vi "ReversedEngineering QueuedStateMachinieMemory.vi"(1 "VIName":string, 2 "StateJumps":string[](array[string]), 5 "error in (no error)":errorcluster, 6 "Action(GetInsertQueuedArrayElementsVI)":T1=enum."GetInsertQueuedArrayElementsVI") -> (15 "StateJumpsOut":string[][](array[string]), 16 "VIName":string, 19 "error out":errorcluster)   [LabVIEW 2020]
uses:
  <resource>/Framework/Providers/Open_GDS/UML/ReversedEngineering/ReversedEngineering QueuedStateMachinMemoryAction.ctl
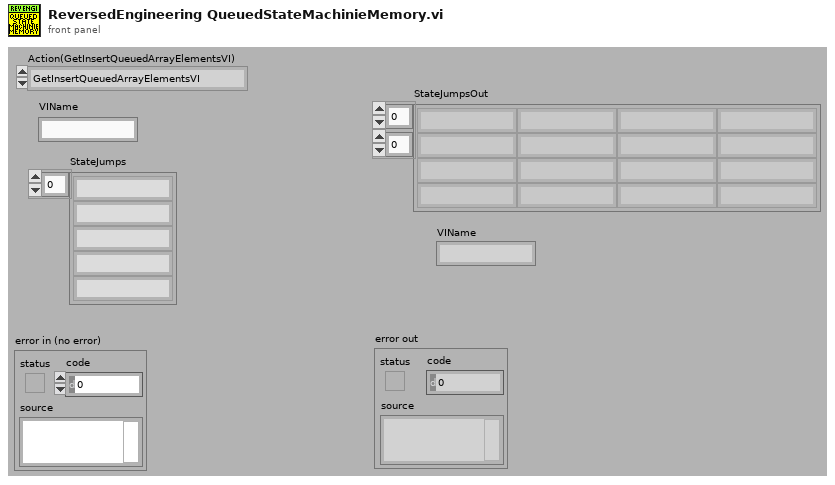
[diagram p1: front panel]
types:
  T1 = typedef "ReversedEngineering QueuedStateMachinMemoryAction.ctl" = enum16{"Initialize", "GetInsertQueuedArrayElementsVI", "SetQueuedStateJumps", "GetQueuedStateJumps"}
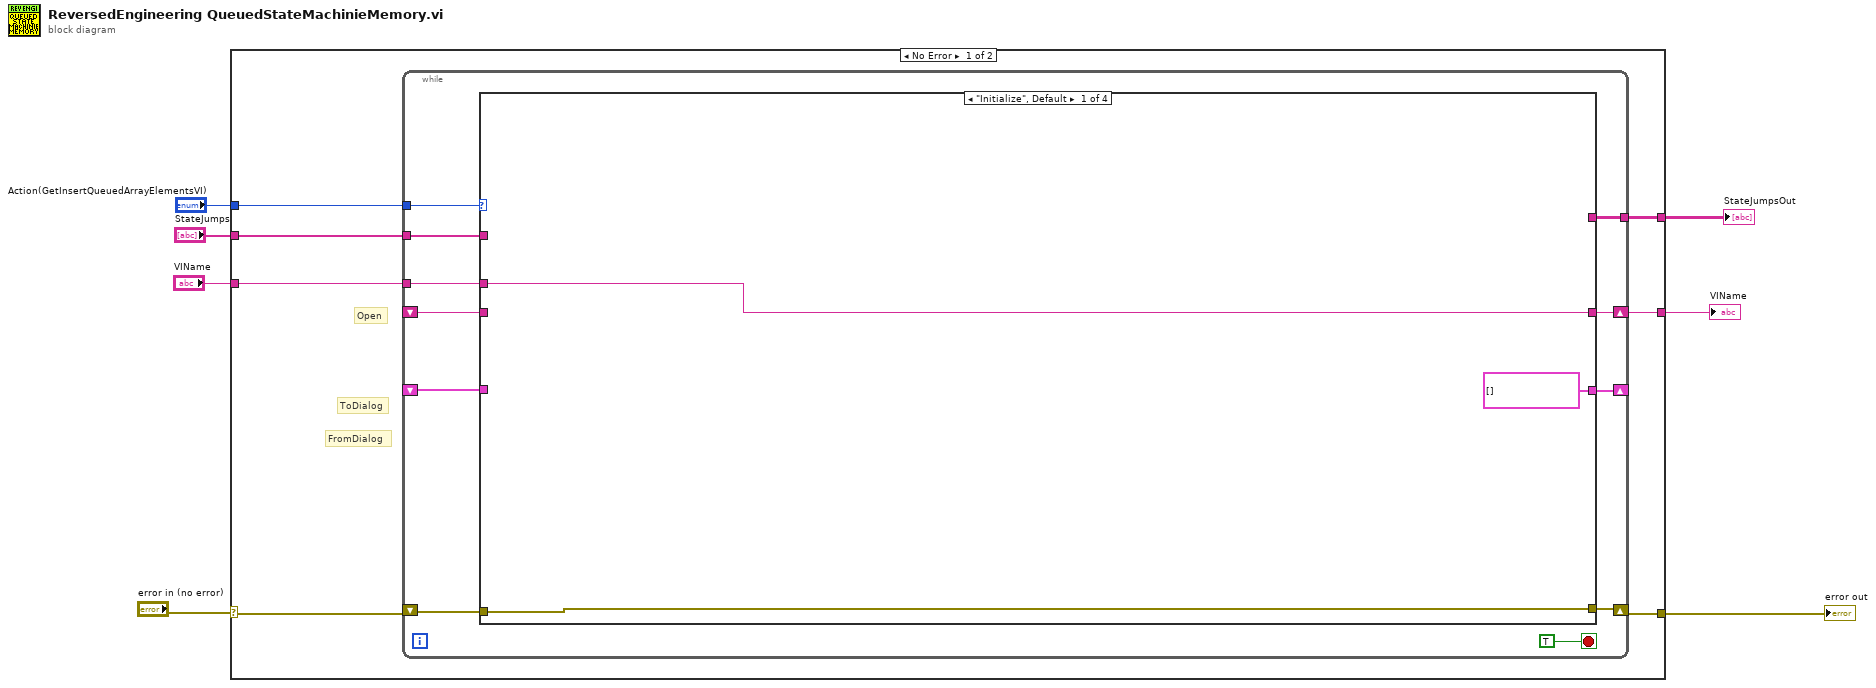
[diagram p0: block diagram]
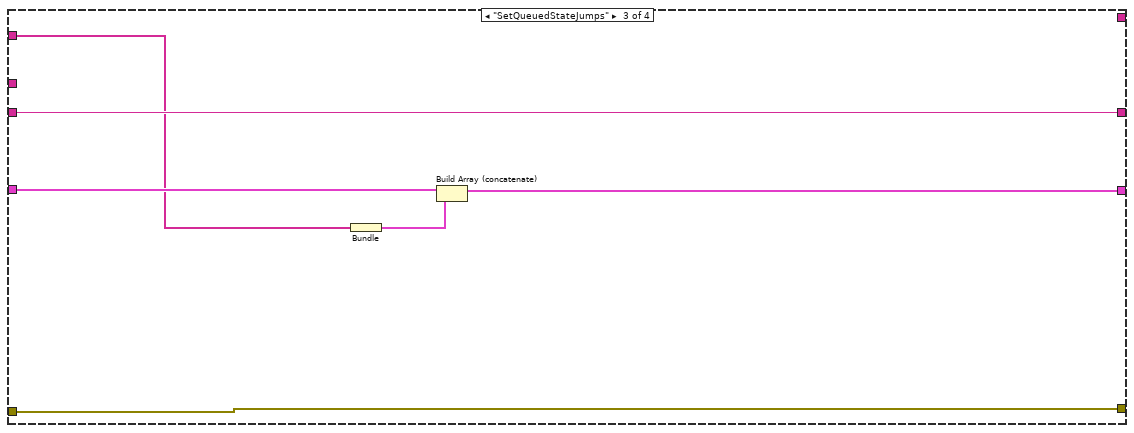
[diagram p3: hidden frame]
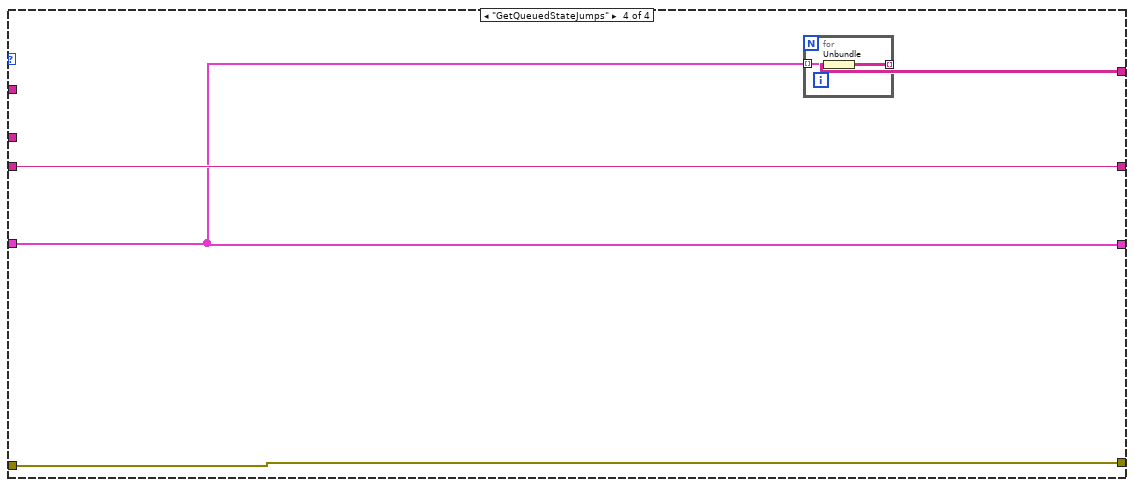
[diagram p4: hidden frame]
diagram:
  n1 = case shown="No Error" "error in (no error)" {
    selector: "error in (no error)" -> [w13 w44]
    tunnel: [w12 w44] -> w1
    tunnel: "Action(GetInsertQueuedArrayElementsVI)" -> [w14 _]
    tunnel: "VIName" -> [w11 _]
    tunnel: [w10 _] -> w4
    tunnel: "StateJumps" -> [w9 _]
    tunnel: [w8 _] -> w2
    frame No Error {
      # "Open"
      # "FromDialog"
      # "ToDialog"
      n2 = while {
        tunnel: w14 -> [w25]
        shift-right: [w23] -> w12
        shift-left: w13 -> [w24]
        tunnel: w11 -> [w21]
        shift-right: [w20] -> w10
        shift-left: _ -> [w19]
        shift-right: [w16] -> _
        shift-left: _ -> [w18]
        tunnel: w9 -> [w17]
        tunnel: [w15] -> w8
        stop <- TRUE stop-if-true
        n3 = case shown="\"Initialize\", Default" w25 {
          tunnel: [w28 w30 w36 w41] -> w23
          tunnel: w24 -> [w28 w30 w36 w41]
          tunnel: w21 -> [w27 _ _ _]
          tunnel: [w27 w31 w37 w39] -> w20
          tunnel: w19 -> [_ w31 w37 w39]
          tunnel: w18 -> [_ w29 w35 w38]
          tunnel: w17 -> [_ _ w33 _]
          tunnel: [cluster{"StateJumps":string[]}[] [] w29 w32 w38] -> w16
          tunnel: [_ _ _ w40] -> w15
          frame "Initialize", Default {
          }
          frame "GetInsertQueuedArrayElementsVI" {
          }
          frame "SetQueuedStateJumps" {
            n4 = Bundle("StateJumps"=w33) -> (w34:cluster{"StateJumps":string[]})  [unwired: 1 in]
            n5 = Build Array (concatenate)(w35, w34) -> (w32:cluster{"StateJumps":string[]}[])
          }
          frame "GetQueuedStateJumps" {
            n6 = for {
              tunnel: w38 -> [w43] mode=indexing
              tunnel: [w42] -> w40 mode=indexing
              n7 = Unbundle(w43) -> ("StateJumps"=w42:string[])
            }
          }
        }
      }
    }
    frame Error {
    }
  }
  "error out" <- w1
  "StateJumpsOut" <- w2
  "VIName" <- w4
